vi "subTiE_SetZPos.vi"(6 "Ref":T2 caption="Ref (can be hidden)", 7 "TI-Ctrl":T1={"Obj"=5, "Cube Bottom"=5, "Cube Top"=1, "PFS-Ctrl"={"PFS IO"=FALSE, "PSF Err"=FALSE, "PSF Pos"=0}, "Z-Ctrl"={"Z-pos"=499.875, "Home"=FALSE, "Sensitivity"=1}, "Condenser"=2, "Lightpath"=enum."EYE"} {"Condenser" items=["A"=1, "DICN2"=2, "- empty 3 -"=3, "- empty 4 -"=4, "- empty 5 -"=5, "- empty 6 -"=6]; "Z-Ctrl"."Sensitivity" min=1 max=3 step=1 scale=1.0..3.0; "PFS-Ctrl"."PSF Pos" scale=0.0..16400.0; "Cube Top" items=["Quad-O"=1, "Quad-R"=2, "empty"=3, "empty"=4, "empty"=5, "DIC"=6]; "Cube Bottom" items=["Cy5"=1, "RFP"=2, "mO2"=3, "empty"=4, "CFP"=5, "GFP"=6]; "Obj" items=["20x/.75 Dry PFS"=1, "40x/1.3 Oil PFS"=2, "60x/1.4 Oil PFS"=3, "- empty 4 -"=4, "- empty 5 -"=5, "- empty 6 -"=6]}, 8 "error in":errorcluster) -> (0 "error out":errorcluster)   [LabVIEW 2015]
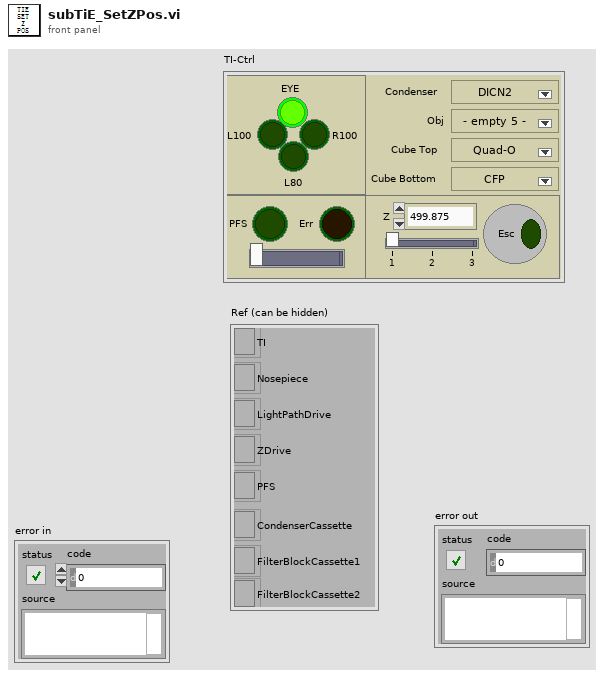
[diagram p1: front panel]
types:
  T1 = cluster{"Obj":u16, "Cube Bottom":u16, "Cube Top":u16, "PFS-Ctrl":cluster{"PFS IO":bool, "PSF Err":bool, "PSF Pos":u32}, "Z-Ctrl":cluster{"Z-pos":dbl, "Home":bool, "Sensitivity":u8}, "Condenser":u16, "Lightpath":enum32{"EYE", "L100", "R100", "L80"}}
  T2 = cluster{"TI":refnum<k7>, "Nosepiece":refnum<k7>, "LightPathDrive":refnum<k7>, "ZDrive":refnum<k7>, "PFS":refnum<k7>, "CondenserCassette":refnum<k7>, "FilterBlockCassette1":refnum<k7>, "FilterBlockCassette2":refnum<k7>}
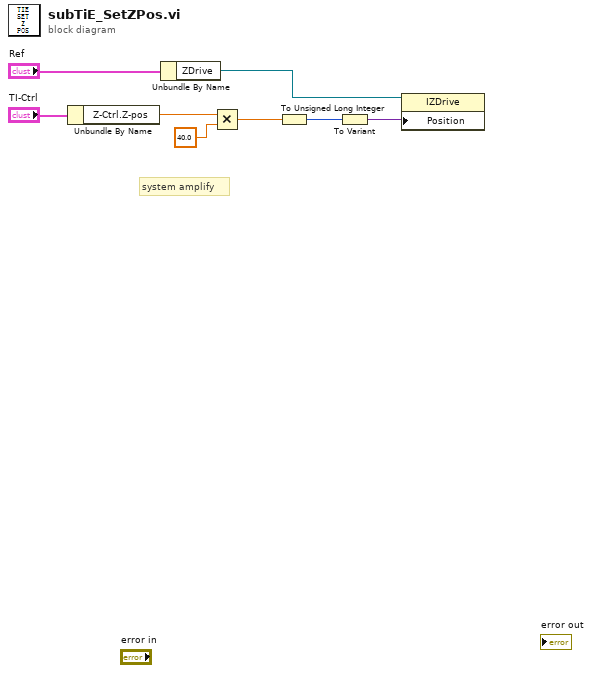
[diagram p0: block diagram]
diagram:
  # "system amplify"
  n1 = Unbundle By Name("TI-Ctrl") -> ("Z-Ctrl.Z-pos"=w7:dbl)
  n2 = Unbundle By Name("Ref") -> ("ZDrive"=w8:refnum<k7>)
  n3 = Multiply(x=w7, y=40.0) -> (x*y=w4:dbl)
  n4 = To Unsigned Long Integer(number=w4) -> (unsigned 32bit integer=w3:u32)
  n5 = To Variant(anything=w3) -> (Variant=w6:variant)
  n6 = property class="IZDrive"(reference=w8, "Position"=w6) -> ()  [unwired: 1 in, 2 out]
